vi "ConfigDevice.vi"(8 "error in (no error)":errorcluster, 11 "ChromaPowerSupplyModel in":refnum<class "ChromaPowerSupplyModel.lvclass">) -> (0 "error out":errorcluster, 3 "ChromaPowerSupplyModel out":refnum<class "ChromaPowerSupplyModel.lvclass">)   [LabVIEW 2018, in "AcPwrPlugins.lvlib" / "ChromaPowerSupplyModel.lvclass"]
doc: "This VI configures all the properties set by the user through the INI file or the Properties Dialog box."
uses:
  ChromaPowerSupplyModel.lvclass
  ChromaPowerSupplyModel.lvclass/ChromaPowerSupplyModel.ctl
  Database/DatabaseBaseClass/DatabaseBaseClass.lvclass
  <vilib>/addons/database/NI_Database_API.lvlib
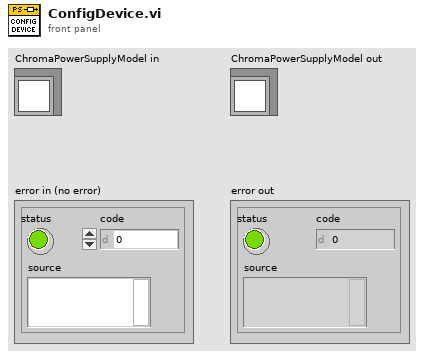
[diagram p1: front panel]
types:
  T1 = typedef "AcPwrPlugins.lvlib/ChromaPowerSupply.lvclass/Device(s)Settings.ctl" = cluster{"Phases":cluster{"Handle":string, "Instrument Options":string, "id query (T)":bool, "reset device (T)":bool, "Timing":cluster{"TimingOn":enum16{""}, "Hours":u32, "Minutes":u32, "Seconds":dbl, "CutoffVoltage":dbl}, "Connected":bool, "Output Mode":enum16{"Voltage (DC)", "Current (DC)"}, "Voltage":dbl, "Current":dbl, "High Voltage Limit":dbl, "High Current Limit":dbl, "Power Protect":dbl, "Current Protect":dbl, "Voltage Protect":dbl, "Low Current Limit":dbl, "Low Voltage Limit":dbl, "Current Slew Rate":dbl, "Voltage Slew Rate":dbl}[], "MeasName":string}
  T2 = typedef "AcPwrPlugins.lvlib/ChromaPowerSupplyModel.lvclass/Database Settings.ctl" = cluster{"Data Source":string, "ICDAS to Model Table":string, "Model to ICDAS Table":string}
  T3 = typedef "NI_Database_API.lvlib/Conn ObjectReference.ctl" = refnum<k1>
  T4 = cluster{"Handle":string, "Instrument Options":string, "id query (T)":bool, "reset device (T)":bool, "Timing":cluster{"TimingOn":enum16{""}, "Hours":u32, "Minutes":u32, "Seconds":dbl, "CutoffVoltage":dbl}, "Connected":bool, "Output Mode":enum16{"Voltage (DC)", "Current (DC)"}, "Voltage":dbl, "Current":dbl, "High Voltage Limit":dbl, "High Current Limit":dbl, "Power Protect":dbl, "Current Protect":dbl, "Voltage Protect":dbl, "Low Current Limit":dbl, "Low Voltage Limit":dbl, "Current Slew Rate":dbl, "Voltage Slew Rate":dbl}[]
  T5 = cluster{"Handle":string, "Instrument Options":string, "id query (T)":bool, "reset device (T)":bool, "Timing":cluster{"TimingOn":enum16{""}, "Hours":u32, "Minutes":u32, "Seconds":dbl, "CutoffVoltage":dbl}, "Connected":bool, "Output Mode":enum16{"Voltage (DC)", "Current (DC)"}, "Voltage":dbl, "Current":dbl, "High Voltage Limit":dbl, "High Current Limit":dbl, "Power Protect":dbl, "Current Protect":dbl, "Voltage Protect":dbl, "Low Current Limit":dbl, "Low Voltage Limit":dbl, "Current Slew Rate":dbl, "Voltage Slew Rate":dbl}
  T6 = cluster{string, "Current":dbl, "Low Current Limit":dbl, "High Current Limit":dbl, "Current Protect":dbl, "Current Slew Rate":dbl, "Voltage":dbl, "Low Voltage Limit":dbl, "High Voltage Limit":dbl, "Voltage Protect":dbl, "Voltage Slew Rate":dbl, "Power Protect":dbl, "seconds since 1Jan1904":timestamp, bool, "current time":timestamp, "Measurement Refresh Time (ms)":u32}
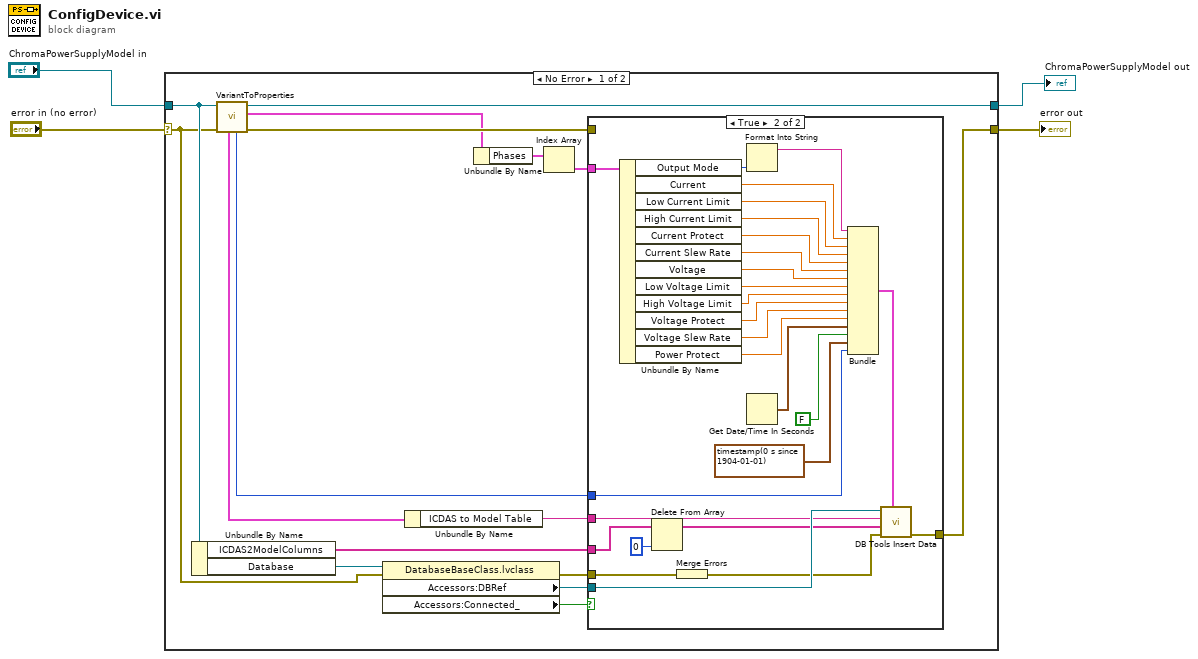
[diagram p0: block diagram]
diagram:
  n1 = case shown="No Error" "error in (no error)" {
    selector: "error in (no error)" -> [w6 w49]
    tunnel: "ChromaPowerSupplyModel in" -> [w17 w50]
    tunnel: [w19 w50] -> w2
    tunnel: [w20 w49] -> w1
    frame No Error {
      n2 = Unbundle By Name(w17) -> ("ICDAS2ModelColumns"=w5:string[], "Database"=w18:refnum<class "DatabaseBaseClass.lvclass">)
      n3 = call "VariantToProperties.vi"("error in (no error)"=w6, "ChromaPowerSupplyModel in"=w17) -> ("error out"=w13:errorcluster, "Device Settings"=w10:T1, "ChromaPowerSupplyModel out"=w19:refnum<class "ChromaPowerSupplyModel.lvclass">, "Measurement Refresh Time (ms)"=w7:u32, "Database Settings"=w12:T2)  [unwired: 4 in, 1 out]
      n4 = property class="DatabaseBaseClass.lvclass"(reference=w18, error in=w6) -> (error out=w16:errorcluster, "Accessors:DBRef"=w14:T3, "Accessors:Connected_"=w15:bool)  [unwired: 1 out]
      n5 = Unbundle By Name(w12) -> ("ICDAS to Model Table"=w11:string)
      n6 = Unbundle By Name(w10) -> ("Phases"=w9:T4)
      n7 = Index Array(array=w9) -> (element=w8:T5)  [unwired: 1 in]
      n8 = case shown="True" w15 {
        tunnel: [w21 w48] -> w20
        tunnel: w16 -> [_ w47]
        tunnel: w14 -> [_ w46]
        tunnel: w13 -> [w21 _]
        tunnel: w11 -> [_ w44]
        tunnel: w8 -> [_ w42]
        tunnel: w7 -> [_ w22]
        tunnel: w5 -> [_ w34]
        frame False {
        }
        frame True {
          n9 = Unbundle By Name(w42) -> ("Output Mode"=w31:enum16{"Voltage (DC)", "Current (DC)"}, "Current"=w35:dbl, "Low Current Limit"=w36:dbl, "High Current Limit"=w37:dbl, "Current Protect"=w38:dbl, "Current Slew Rate"=w39:dbl, "Voltage"=w40:dbl, "Low Voltage Limit"=w41:dbl, "High Voltage Limit"=w29:dbl, "Voltage Protect"=w28:dbl, "Voltage Slew Rate"=w27:dbl, "Power Protect"=w26:dbl)
          n10 = Delete From Array(array=w34, index=0) -> (array with subset deleted=w32:string[])  [unwired: 1 in, 1 out]
          n11 = Merge Errors(w47) -> (w45:errorcluster)
          n12 = Format Into String(w31) -> (resulting string=w30:string)  [unwired: 3 in, 1 out]
          n13 = Get Date/Time In Seconds() -> (seconds since 1Jan1904=w25:timestamp)
          n14 = Bundle(w30, "Current"=w35, "Low Current Limit"=w36, "High Current Limit"=w37, "Current Protect"=w38, "Current Slew Rate"=w39, "Voltage"=w40, "Low Voltage Limit"=w41, "High Voltage Limit"=w29, "Voltage Protect"=w28, "Voltage Slew Rate"=w27, "Power Protect"=w26, "seconds since 1Jan1904"=w25, FALSE, "current time"=timestamp(0 s since 1904-01-01), "Measurement Refresh Time (ms)"=w22) -> (w43:T6)  [unwired: 1 in]
          n15 = call <vilib>:"DB Tools Insert Data.vi"("data"=w43, "error in (no error)"=w45, "columns"=w32, "table"=w44, "connection reference"=w46) -> ("error out"=w48:errorcluster)  [unwired: 5 in, 1 out]
        }
      }
    }
    frame Error {
    }
  }
  "error out" <- w1
  "ChromaPowerSupplyModel out" <- w2
